vi "GenerateUniqueFilename.vi"(5 "Index digits":i32=3, 6 "No index opion":string, 7 "format string":string, 8 "Error In":errorcluster, 9 "File name suffixes":string[](array[string]), 10 "File name prefix":string, 11 "Folder Path Control":path) -> (0 "Error Out":errorcluster, 3 "Paths":path[](array[path]))   [LabVIEW 2016]
panel:
  out "Any file exists?":bool
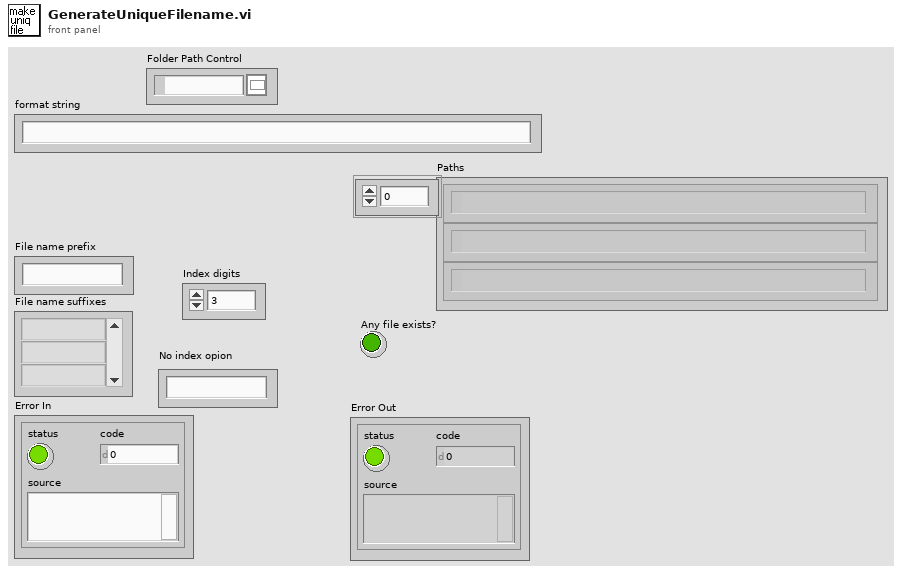
[diagram p1: front panel]
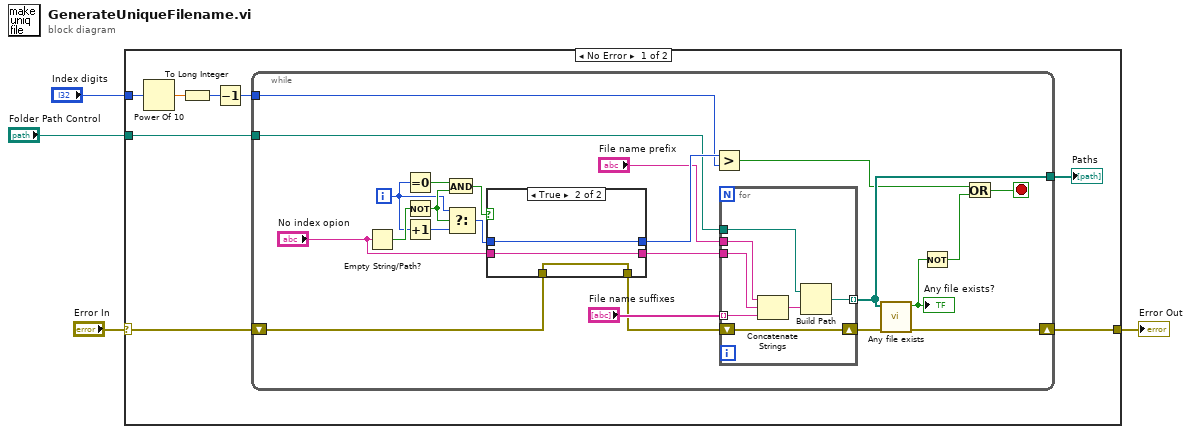
[diagram p0: block diagram]
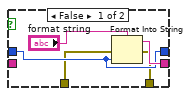
[diagram p2: hidden frame]
diagram:
  n1 = case shown="No Error" "Error In" {
    selector: "Error In" -> [w11 w51]
    tunnel: [w12 w51] -> w3
    tunnel: "Index digits" -> [w9 _]
    tunnel: "Folder Path Control" -> [w5 _]
    frame No Error {
      n2 = Power Of 10(x=w9) -> (10^x=w8:dbl)
      n3 = To Long Integer(number=w8) -> (32bit integer=w7:i32)
      n4 = Decrement(x=w7) -> (x-1=w6:i32)
      n5 = while {
        tunnel: [w32] -> w10
        shift-right: [w27] -> w12
        shift-left: w11 -> [w14]
        tunnel: w6 -> [w18]
        tunnel: w5 -> [w17]
        i -> [w20]
        stop <- w33 stop-if-true
        n6 = Empty String/Path?(string/path="No index opion") -> (empty?=w25:bool)
        n7 = Equal To 0?(x=w20) -> (x = 0?=w22:bool)
        n8 = Not(x=w25) -> (.not. x?=w21:bool)
        n9 = Increment(x=w20) -> (x+1=w19:i32)
        n10 = And(x=w22, y=w21) -> (x .and. y?=w24:bool)
        n11 = Select(t=w20, s=w21, f=w19) -> (s? t:f=w26:i32)
        n12 = case shown="True" w24 {
          tunnel: [w40 w42] -> w35
          tunnel: [w38 w43] -> w34
          tunnel: w26 -> [w38 w43]
          tunnel: "No index opion" -> [_ w42]
          tunnel: w14 -> [w37 w41]
          tunnel: [w36 w41] -> w13
          frame False {
            n13 = Format Into String(format string="format string", error in=w37, w38) -> (resulting string=w40:string, error out=w36:errorcluster)  [unwired: 1 in]
          }
          frame True {
          }
        }
        n14 = Greater?(x=w34, y=w18) -> (0:w15:bool)
        n15 = for {
          tunnel: w35 -> [w50]
          tunnel: [w44] -> w32 mode=indexing
          tunnel: "File name suffixes" -> [w49] mode=indexing
          shift-right: [w48] -> w28
          shift-left: w13 -> [w48]
          tunnel: "File name prefix" -> [w47]
          tunnel: w17 -> [w46]
          n16 = Concatenate Strings(w47, w50, w49) -> (w45:string)
          n17 = Build Path(base path=w46, name or relative path=w45) -> (appended path=w44:path)
        }
        n18 = call "Any file exists.vi"("Error In"=w28, "Files"=w32) -> ("Error Out"=w27:errorcluster, "Any file exists?"=w31:bool)  [unwired: 8 in]
        "Any file exists?" <- w31
        n19 = Not(x=w31) -> (.not. x?=w16:bool)
        n20 = Or(x=w15, y=w16) -> (x .or. y?=w33:bool)
      }
      "Paths" <- w10
    }
    frame Error {
    }
  }
  "Error Out" <- w3
